vi "test Desired Speed.vi"(8 "error in (no error)":errorcluster, 11 "TestCase in":refnum<class "Engine Simulation IO System Tests.lvclass">) -> (0 "error out":errorcluster, 3 "TestCase out":refnum<class "Engine Simulation IO System Tests.lvclass">)   [LabVIEW 2017, in "Engine Simulation IO System Tests.lvclass"]
uses:
  Engine Simulation IO System Tests.lvclass
  C:/github/niveristand-custom-device-testing-tools/VeriStandTestCase/VeriStandTestCase.lvclass
  <vilib>/NI Veristand/Execution/Workspace/NI VeriStand - Set Single Channel Value.vi
  <vilib>/NI Veristand/Execution/Workspace/NI VeriStand - Get Single Channel Value.vi
  <vilib>/addons/_JKI Toolkits/VI Tester/TestCase.llb/TestCase.lvclass
  <vilib>/NI VeriStand/Execution/Workspace/NI_VS Workspace ExecutionAPI.lvlib
  C:/Program Files (x86)/National Instruments/LabVIEW 2017/vi.lib/addons/_JKI Toolkits/VI Tester/TestCase.llb/TestCase.lvclass
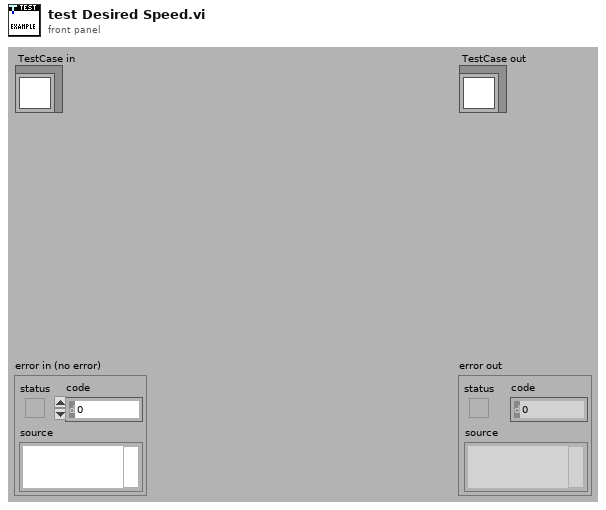
[diagram p1: front panel]
types:
  T1 = typedef "NI_VS Workspace ExecutionAPI.lvlib/WorkspaceAPI.ctl" = refnum<k24>
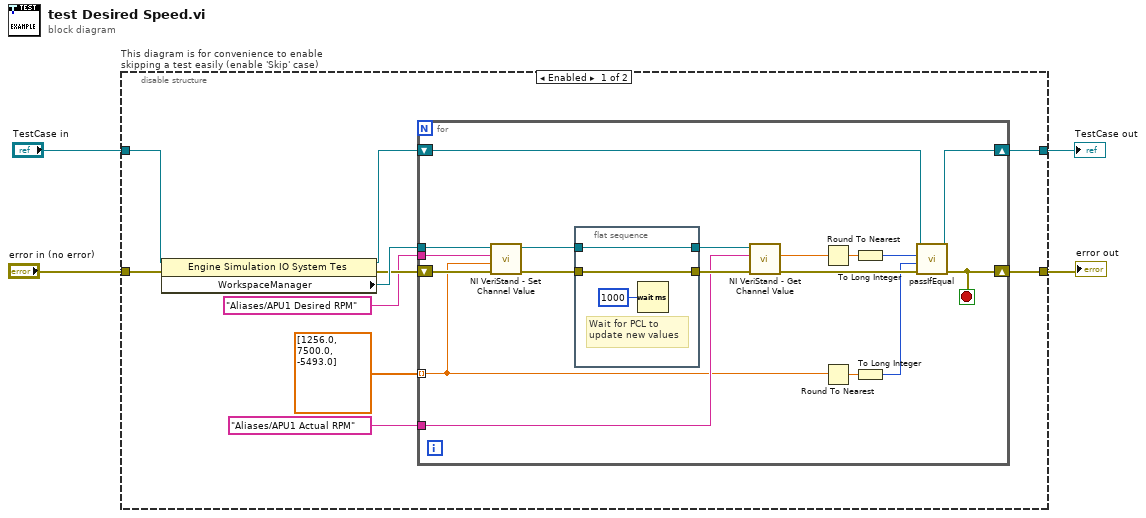
[diagram p0: block diagram]
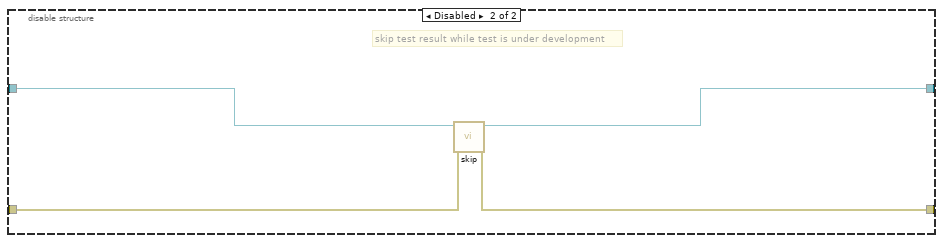
[diagram p2: hidden frame]
diagram:
  n1 = disable-structure "This diagram is for convenience to enable skipping a test easily (enable 'Skip' case)" shown="Enabled" {
    disable-tunnel: "TestCase in" -> [w11 w39]
    disable-tunnel: [w5 w37] -> w1
    disable-tunnel: [w9 w38] -> w3
    disable-tunnel: "error in (no error)" -> [w10 w36]
    frame Enabled {
      n2 = property class="Engine Simulation IO System Tes"(reference=w11, error in=w10) -> (reference out=w6:refnum<class "Engine Simulation IO System Tests.lvclass">, error out=w13:errorcluster, "WorkspaceManager"=w14:T1)
      n3 = for {
        tunnel: w14 -> [w32]
        tunnel: "Aliases/APU1 Desired RPM" ("Channel") -> [w30]
        shift-right: [w15] -> w9
        shift-left: w13 -> [w31]
        tunnel: dbl[] [1256.0, 7500.0, -5493.0] -> [w21] mode=indexing
        tunnel: "Aliases/APU1 Actual RPM" ("Channel") -> [w25]
        shift-right: [w16] -> w5
        shift-left: w6 -> [w17]
        stop <- w15 stop-if-true
        n4 = call-poly <vilib>:"NI VeriStand - Set Channel Value.vi"("error in (no error)"=w31, "Value"=w21, "Channel"=w30, "WorkspaceManager in"=w32) -> ("error out"=w29:errorcluster, "WorkspaceManager out"=w28:T1)  [unwired: 6 in]
        n5 = flat-sequence {
          tunnel: w28 -> [w34]
          tunnel: w29 -> [w35]
          tunnel: [w35] -> w27
          tunnel: [w34] -> w26
          frame #0 {
            # "Wait for PCL to\nupdate new values"
            n6 = Wait (ms)(milliseconds to wait=u32 1000) -> ()  [unwired: 1 out]
          }
        }
        n7 = call-poly <vilib>:"NI VeriStand - Get Channel Value.vi"("error in (no error)"=w27, "Channel"=w25, "WorkspaceManager in"=w26) -> ("error out"=w20:errorcluster, "Value"=w22:dbl)  [unwired: 6 in, 1 out]
        n8 = Round To Nearest(number=w22) -> (nearest integer value=w24:dbl)
        n9 = Round To Nearest(number=w21) -> (nearest integer value=w23:dbl)
        n10 = To Long Integer(number=w24) -> (32bit integer=w19:i32)
        n11 = To Long Integer(number=w23) -> (32bit integer=w18:i32)
        n12 = call-dynamic "passIfEqual.vi"("error in (no error)"=w20, "y"=w18, "x"=w19, "TestCase in"=w17) -> ("error out"=w15:errorcluster, "TestCase out"=w16:refnum<class "Engine Simulation IO System Tests.lvclass">)  [unwired: 6 in]
      }
    }
    frame Disabled {
      # "skip test result while test is under development"
      n13 = call <vilib>:"skip.vi"("error in (no error)"=w36, "TestCase in"=w39) -> ("error out"=w38:errorcluster, "TestCase out"=w37:refnum<class "Engine Simulation IO System Tests.lvclass">)  [unwired: 8 in]
    }
  }
  "error out" <- w3
  "TestCase out" <- w1
